vi "Read Measurement (Histogram).vi"(0 "VISA resource name":refnum<visa-resource-name>, 7 "Histogram Function (0: Histogram Hits)":i32(ring) items=["Histogram Hits", "Histogram M1S", "Histogram M2S", "Histogram M3S", "Histogram Max", "Histogram Mean", "Histogram Median", "Histogram Min", "Histogram Peak", "Histogram P-P", "Histogram Std Dev", "Histogram Resolution", "Histogram Mode"], 9 "Maximum Time (10000ms)":u32=10000, 11 "error in (no error)":errorcluster) -> (4 "VISA resource name out":refnum<visa-resource-name>, 6 "Measurement":dbl, 15 "error out":errorcluster)   [LabVIEW 2020, in "Agilent 90000 Series.lvlib"]
doc: "Initiates an acquisition on Histogram that you enable with the Configure Histogram VI. It then waits for the acquisition to complete, obtains a Histogram measurement on the channel you specify, and returns the measurement value. You specify a Histogram measurement type, such as Hits, Min and Max.You can call the Fetch Measurement (Histogram).vi separately for any other waveform measurement that you want to obtain on a specific channel without initiating another acquisition."
uses:
  Agilent 90000 Series.lvlib
  Low Level/Fetch Measurement (Histogram).vi
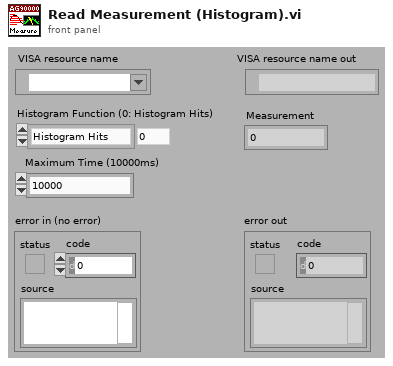
[diagram p1: front panel]
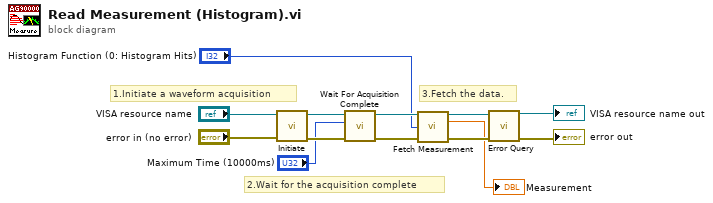
[diagram p0: block diagram]
diagram:
  # "3.Fetch the data."
  # "2.Wait for the acquisition complete"
  # "1.Initiate a waveform acquisition"
  n1 = call "Initiate.vi"("error in (no error)"="error in (no error)", "VISA resource name"="VISA resource name") -> ("error out"=w6:errorcluster, "VISA resource name out"=w7:refnum<visa-resource-name>)  [unwired: 8 out]
  n2 = call "Wait For Acquisition Complete.vi"("error in (no error)"=w6, "Maximum Time (10000ms)"="Maximum Time (10000ms)", "VISA resource name"=w7) -> ("error out"=w9:errorcluster, "VISA resource name out"=w8:refnum<visa-resource-name>)  [unwired: 7 out]
  n3 = call-poly "Fetch Measurement.vi"("VISA resource name"=w8, "Histogram Function (0: Histogram Hits)"="Histogram Function (0: Histogram Hits)", "error in (no error)"=w9) -> ("VISA resource name out"=w5:refnum<visa-resource-name>, "Measurement"=→"Measurement":dbl, "error out"=w4:errorcluster)  [unwired: 10 out]
  n4 = call "Error Query.vi"("error in (no error)"=w4, "VISA resource name"=w5) -> ("error out"=→"error out":errorcluster, "VISA resource name out"=→"VISA resource name out":refnum<visa-resource-name>)  [unwired: 8 out]
